vi "CRYPIC LOG OUT.vi"(8 "pVIRef":refnum<vi>, 10 "sData":string) -> ()   [LabVIEW 2013]
uses:
  CRYMain Sub Window Global.vi
  CRYProject/CRYProject Editor Global.vi
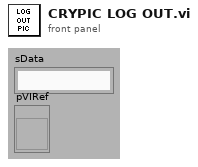
[diagram p1: front panel]
types:
  T1 = enum16{"open", "open or create", "create or replace", "create", "open (read only)"}
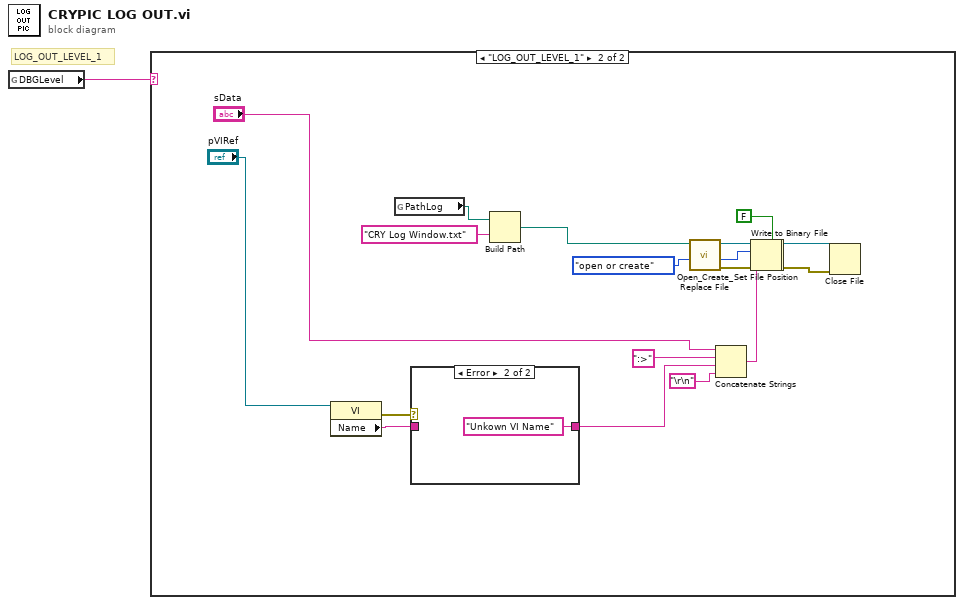
[diagram p0: block diagram]
diagram:
  # "LOG_OUT_LEVEL_1"
  n1 = global read "CRYMain Sub Window Global.vi" "DBGLevel"() -> (w1:string)
  n2 = case shown="\"LOG_OUT_LEVEL_1\"" w1 {
    frame Default {
    }
    frame "LOG_OUT_LEVEL_1" {
      n3 = property class="VI"(reference="pVIRef") -> (error out=w7:errorcluster, "Name"=w6:string)  [unwired: 1 in, 1 out]
      n4 = global read "CRYProject Editor Global.vi" "PathLog"() -> (w2:path)
      n5 = case shown="Error" w7 {
        tunnel: w6 -> [w22 _]
        tunnel: [w22 "Unkown VI Name" ("Name")] -> w4
        frame No Error {
        }
        frame Error {
        }
      }
      n6 = Build Path(base path=w2, name or relative path="CRY Log Window.txt" ("name")) -> (appended path=w10:path)
      n7 = call <vilib>:"Open_Create_Replace File.vi"("function (open:0)"=T1."open or create", "file path"=w10) -> ("error out"=w19:errorcluster, "file size (bytes)"=w17:i32, "refnum"=w18:refnum<file>)  [unwired: 6 in, 1 out]
      n8 = Concatenate Strings("sData", ":>" ("string"), w4, "\r\n") -> (w14:string)
      n9 = Set File Position(offset (in bytes) (0)=w17, refnum=w18, error in=w19) -> (refnum out=w13:refnum<file>, error out=w12:errorcluster)  [unwired: 1 in]
      n10 = Write to Binary File(file (use dialog)=w13, data=w14, error in=w12, 5:FALSE ("prepend array or string size? (T)")) -> (refnum out=w15:refnum<file>, error out=w16:errorcluster)  [unwired: 2 in, 1 out]
      n11 = Close File(refnum=w15, error in=w16) -> ()  [unwired: 2 out]
    }
  }
